vi "is valid.vi"(11 "connection in":refnum<class "TCP connection.lvclass">) -> (3 "valid":bool)   [LabVIEW 2015, in "TCP connection.lvclass"]
uses:
  TCP connection.lvclass
  TCP connection.lvclass/TCP connection.ctl
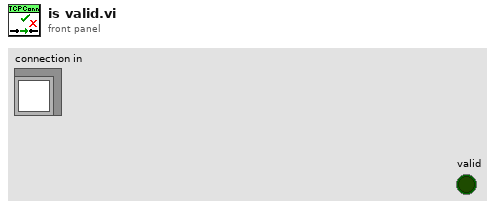
[diagram p1: front panel]
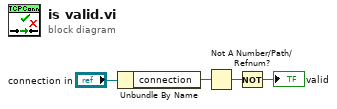
[diagram p0: block diagram]
diagram:
  n1 = Unbundle By Name("connection in") -> ("connection"=w2:refnum<k5>)
  n2 = Not A Number/Path/Refnum?(number/path/refnum=w2) -> (NaN/Path/Refnum?=w4:bool)
  n3 = Not(x=w4) -> (.not. x?=→"valid":bool)
